vi "Cauchy CDF.vi"(9 "b":dbl=1.0, 10 "a":dbl, 11 "x":dbl) -> (0 "error":i32, 3 "cdf(x)":dbl=0.5)   [LabVIEW 2017, in "NI_Gmath.lvlib"]
doc: "Computes the continuous cumulative distribution function (CDF), or the probability that the random variate X, where X describes the selected distribution type, has a value less than or equal to <B>x</B>. You must manually select the polymorphic instance to use."
uses:
  NI_Gmath.lvlib
  st_error_code.ctl
panel:
  # "Cauchy CDF"
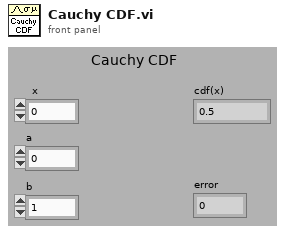
[diagram p1: front panel]
types:
  T1 = typedef "NI_Gmath.lvlib/st_error_code.ctl" = i32
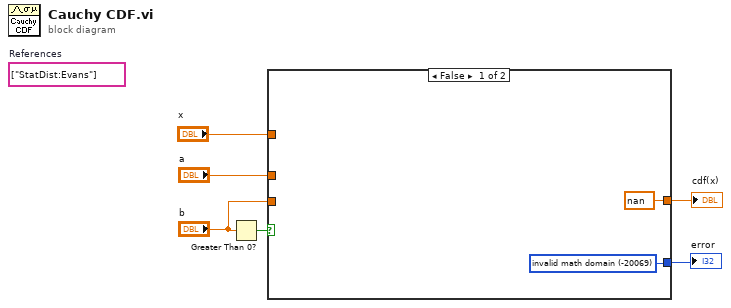
[diagram p0: block diagram]
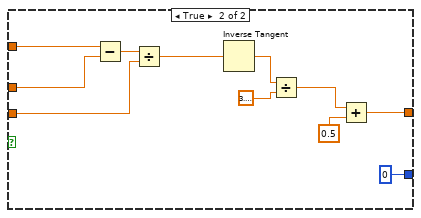
[diagram p2: hidden frame]
diagram:
  (unwired) string[] ["StatDist:Evans"]  # References
  n1 = Greater Than 0?(x="b") -> (x > 0?=w1:bool)
  n2 = case shown="False" w1 {
    tunnel: "b" -> [_ w15]
    tunnel: [w7 0 ("invalid math domain")] -> w6
    tunnel: [nan w9] -> w5
    tunnel: "x" -> [_ w18]
    tunnel: "a" -> [_ w17]
    frame False {
      w7 = T1 -20069 items=["invalid math domain"=-20069, "Fourier interpolation size m >= n"=-20070, "empty array"=-20003] ("stat interp error code")
    }
    frame True {
      n3 = Subtract(x=w18, y=w17) -> (x-y=w16:dbl)
      n4 = Divide(x=w16, y=w15) -> (x/y=w13:dbl)
      n5 = Inverse Tangent(1:w13) -> (0:w12:dbl)
      n6 = Divide(x=w12, y=3.141592653589793) -> (x/y=w10:dbl)
      n7 = Add(x=w10, y=0.5 ("x")) -> (x+y=w9:dbl)
    }
  }
  "cdf(x)" <- w5
  "error" <- w6
